vi "MeasureLCR.vi"(0 "Input parameters":T1={"Measurement type"=enum."Test", "Sensor type"=enum."HPK_8in_256", "Identifier"="test.txt", "Open after execution?"=FALSE, "Plot after execution?"=FALSE, "Display channel"=0, "Voltage Delay (s)"=0.5, "Switch Delay (s)"=0.01, "VISA resource name source"="", "VISA resource name DMM"="", "VISA resource name LCR"="", "Compliance  Level (uA)"=10.0, "Voltage Limit (V)"=1000.0, "Data storage location"="", "Scan voltages"="", "Use source as DMM?"=FALSE, "Single channel?"=FALSE, "LCR signal frequenzy (Hz)"=10.0, "DMM device"=enum."Keithley2001", "Sampling number"=1, "Use env. sensors on"=enum."Sensirion sht1x/7x", "Switchboard Handle"=0, "Use Switchboard"=FALSE, "LCR signal voltage (V)"=10000.0, "Repeat"=1} {"Voltage Limit (V)" format="%#_13g"; "Voltage Delay (s)" format="%#_13g"; "Switch Delay (s)" format="%#_13g"}, 5 "Frequency (Hz)":dbl=10000.0, 11 "error in (no error)":errorcluster) -> (2 "Cp error [pF]":dbl, 3 "Cs error [pF]":dbl, 4 "Cp [pF]":dbl, 6 "Cs [pF]":dbl, 8 "Z (impedance)":dbl, 10 "Theta (Phase)":dbl, 13 "Theta error":dbl, 14 "Z error":dbl, 15 "error out":errorcluster)   [LabVIEW 2016]
uses:
  Input_parameters.ctl
  instr.lib/Agilent E4980/Agilent E4980.lvlib
  <vilib>/Analysis/NI_AALBase.lvlib
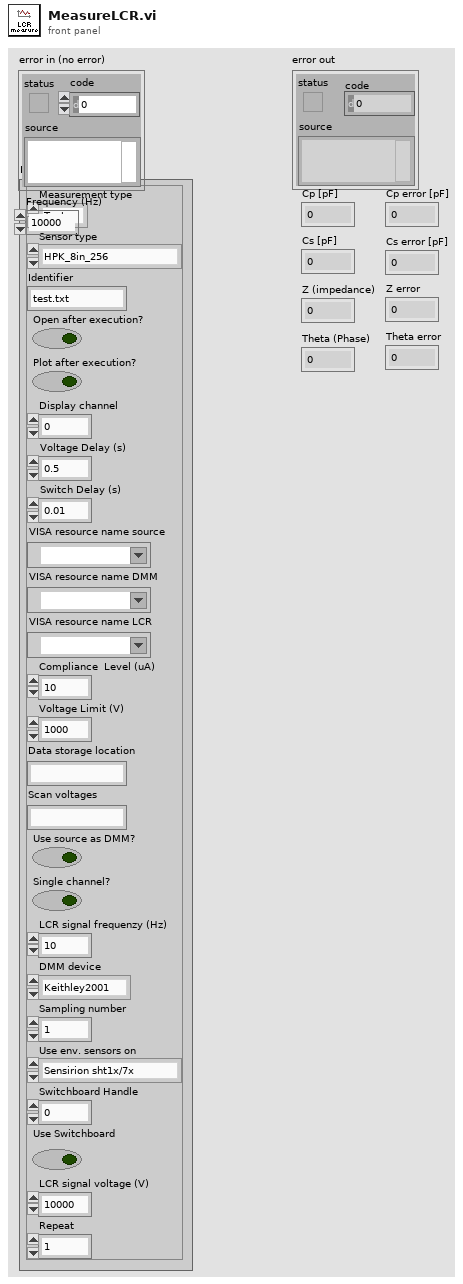
[diagram p1: front panel]
types:
  T1 = typedef "Input_parameters.ctl" = cluster{"Measurement type":enum16{"IV", "CV", "Test"}, "Sensor type":enum16{"HPK_6in_135", "HPK_8in_256", "INF_8in_256", "Diode", "HPK_6in_256", "Test capacitances"}, "Identifier":string, "Open after execution?":bool, "Plot after execution?":bool, "Display channel":i32, "Voltage Delay (s)":dbl, "Switch Delay (s)":dbl, "VISA resource name source":refnum<visa-resource-name>, "VISA resource name DMM":refnum<visa-resource-name>, "VISA resource name LCR":refnum<visa-resource-name>, "Compliance  Level (uA)":dbl, "Voltage Limit (V)":dbl, "Data storage location":string, "Scan voltages":string, "Use source as DMM?":bool, "Single channel?":bool, "LCR signal frequenzy (Hz)":dbl, "DMM device":enum16{"Keithley2001", "Keithley2450", "Keithley2410", "Keithley6487"}, "Sampling number":i32, "Use env. sensors on":enum16{"Sensirion sht1x/7x", "Switch Matrix", "Probecard"}, "Switchboard Handle":u32, "Use Switchboard":bool, "LCR signal voltage (V)":dbl, "Repeat":i32}
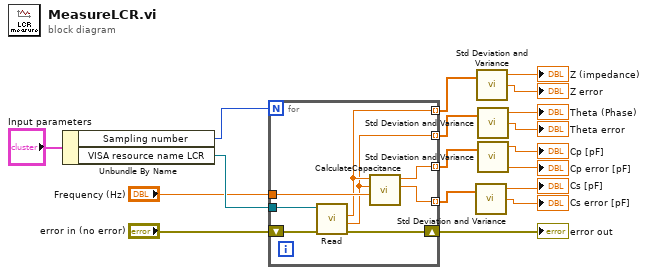
[diagram p0: block diagram]
diagram:
  n1 = Unbundle By Name("Input parameters") -> ("Sampling number"=w13:i32, "VISA resource name LCR"=w16:refnum<visa-resource-name>)
  n2 = for {
    N: w13 -> [_]
    tunnel: w16 -> [w25]
    tunnel: "Frequency (Hz)" -> [w23]
    tunnel: [w22] -> w8 mode=indexing
    tunnel: [w21] -> w3 mode=indexing
    tunnel: [w20] -> w11 mode=indexing
    tunnel: [w19] -> w10 mode=indexing
    shift-right: [w26] -> w17
    shift-left: "error in (no error)" -> [w24]
    n3 = call "Read.vi"("error in (no error)"=w24, "VISA resource name"=w25) -> ("error out"=w26:errorcluster, "Secondary Parameter"=w19:dbl, "Primary Parameter"=w20:dbl)  [unwired: 6 in, 1 out]
    n4 = call "CalculateCapacitance.vi"("Frequency (Hz)"=w23, "Theta (Phase)"=w19, "Z (impedance)"=w20) -> ("Cs [pF]"=w21:dbl, "Cp [pF]"=w22:dbl)  [unwired: 7 in]
  }
  "error out" <- w17
  n5 = call <vilib>:"Std Deviation and Variance.vi"("X"=w3) -> ("mean"=→"Cs [pF]":dbl, "standard deviation"=→"Cs error [pF]":dbl)  [unwired: 1 in, 1 out]
  n6 = call <vilib>:"Std Deviation and Variance.vi"("X"=w11) -> ("mean"=→"Z (impedance)":dbl, "standard deviation"=→"Z error":dbl)  [unwired: 1 in, 1 out]
  n7 = call <vilib>:"Std Deviation and Variance.vi"("X"=w10) -> ("mean"=→"Theta (Phase)":dbl, "standard deviation"=→"Theta error":dbl)  [unwired: 1 in, 1 out]
  n8 = call <vilib>:"Std Deviation and Variance.vi"("X"=w8) -> ("mean"=→"Cp [pF]":dbl, "variance"=→"Cp error [pF]":dbl)  [unwired: 1 in, 1 out]
